vi "GEOM_GetFPA.vi"(8 "error in (no error)":errorcluster, 9 "binned?":bool=TRUE, 10 "readmode":string) -> (0 "error out":errorcluster, 1 "CorrectedFPACoord":T2, 2 "amplifiers":T3[](array[typedef]) {"fliped" items=["none", "horizontal", "vertical"]; "type" items=["LL", "LR", "UL", "UR"]}, 3 "detreadmodes":cluster{"name":string, "detectors":T1[]}, 4 "numyamps":i32, 6 "numxamps":i32)   [LabVIEW 2016]
uses:
  private/vis/GEOM_Amplifier.ctl
  private/vis/GEOM_AmpType.ctl
  private/vis/GEOM_ROI.ctl
  private/vis/GEOM_Coords.ctl
  private/vis/GEOM_CorrectedFPA.ctl
  private/vis/GEOM_DetSummaryStruct.ctl
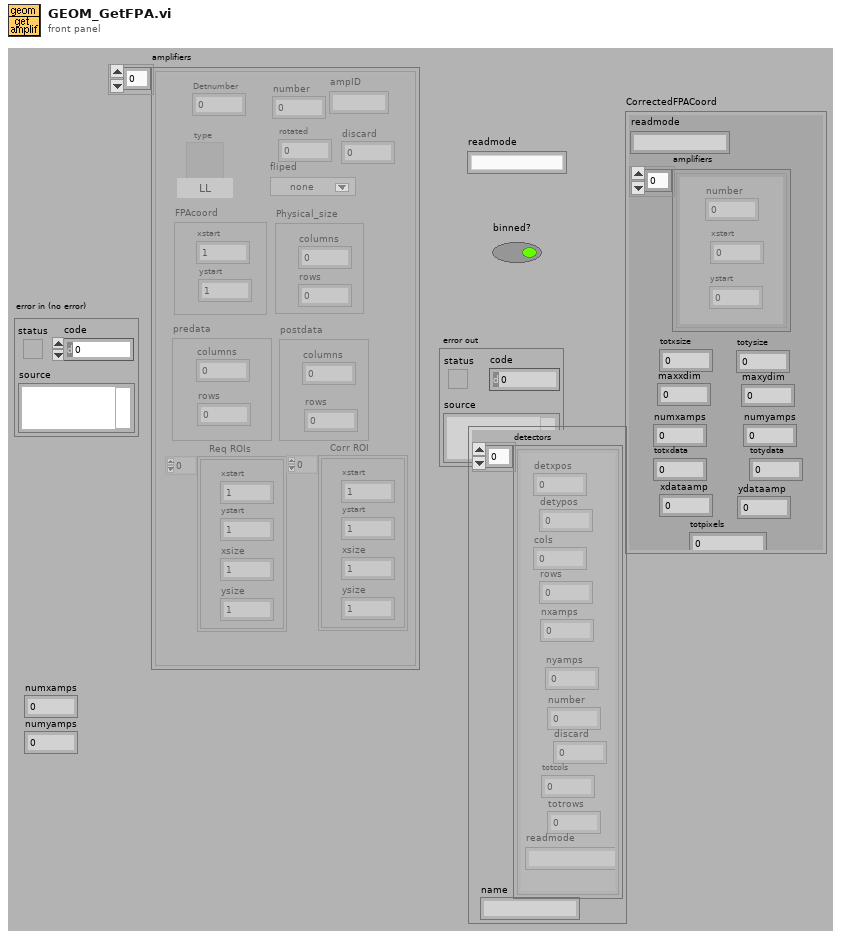
[diagram p1: front panel]
types:
  T1 = typedef "GEOM_DetSummaryStruct.ctl" = cluster{"detxpos":i32, "detypos":i32, "cols":i32, "rows":i32, "nxamps":i32, "nyamps":i32, "number":i32, "discard":i32, "totcols":i32, "totrows":i32, "readmode":string}
  T2 = typedef "GEOM_CorrectedFPA.ctl" = cluster{"readmode":string, "amplifiers":cluster{"number":i32, "xstart":i32, "ystart":i32}[], "totxsize":i32, "totysize":i32, "maxxdim":i32, "maxydim":i32, "numxamps":i32, "numyamps":i32, "totxdata":i32, "totydata":i32, "xdataamp":i32, "ydataamp":i32, "totpixels":i32}
  T3 = typedef "GEOM_Amplifier.ctl" = cluster{"number":i32, "type":T4, "rotated":i16, "fliped":u16, "FPAcoord":cluster{"xstart":i32, "ystart":i32}, "Physical_size":cluster{"columns":i32, "rows":i32}, "predata":cluster{"columns":i32, "rows":i32}, "postdata":cluster{"columns":i32, "rows":i32}, "Req ROIs":T5, "Corr ROI":T5, "Detnumber":i32, "ampID":string, "discard":i32}
  T4 = typedef "GEOM_AmpType.ctl" = u16
  T5 = typedef "GEOM_ROI.ctl" = T6[]
  T6 = typedef "GEOM_Coords.ctl" = cluster{"xstart":u32, "ystart":u32, "xsize":u32, "ysize":u32}
  T7 = cluster{"amplifiers":T3[], "CorrectedFPACoord":T2, "detreadmodes":cluster{"name":string, "detectors":T1[]}}
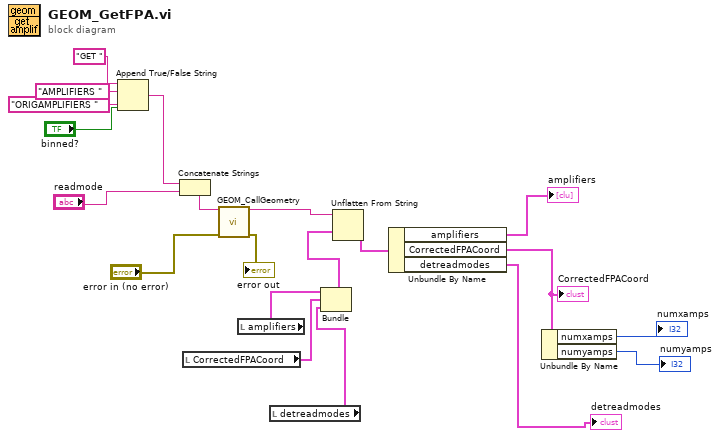
[diagram p0: block diagram]
diagram:
  n1 = Append True/False String(1:"binned?", 2:"ORIGAMPLIFIERS " ("false string"), 3:"AMPLIFIERS " ("true string"), 4:"GET " ("string (\"\")")) -> (0:w6:string)
  n2 = Concatenate Strings(w6, "readmode") -> (w20:string)
  n3 = local read "CorrectedFPACoord"() -> (w14:T2)
  n4 = call "GEOM_CallGeometry.vi"("Command"=w20, "error in (no error)"="error in (no error)") -> ("ImmedReplyString"=w19:string, "error out"=→"error out":errorcluster)  [unwired: 12 out]
  n5 = local read "amplifiers"() -> (w15:T3[])
  n6 = local read "detreadmodes"() -> (w2:cluster{"name":string, "detectors":T1[]})
  n7 = Bundle("amplifiers"=w15, "CorrectedFPACoord"=w14, "detreadmodes"=w2) -> (w13:T7)  [unwired: 1 out]
  n8 = Unflatten From String(type=w13, binary string=w19) -> (value=w12:T7)  [unwired: 1 in, 4 out]
  n9 = Unbundle By Name(w12) -> ("amplifiers"=→"amplifiers":T3[], "CorrectedFPACoord"=w5:T2, "detreadmodes"=→"detreadmodes":cluster{"name":string, "detectors":T1[]})
  "CorrectedFPACoord" <- w5
  n10 = Unbundle By Name(w5) -> ("numxamps"=→"numxamps":i32, "numyamps"=→"numyamps":i32)
